vi "Configure Channel.vi"(0 "KS EDU-X 1002G in":refnum<class "KS EDU-X 1002G.lvclass">, 1 "Vertical Scale (5.0 V)":dbl=5.0, 2 "Enable Channel (True)":bool=TRUE, 3 "Impedance (0: 1 MOhm)":i32(ring) items=["1 MOhm", "50 Ohm"], 5 "Cluster":T1={"Channel (0: Channel 1)"=0, "Vertical Coupling (1: DC)"=1, "Probe Attenuation (10: 10X)"=10, "Vertical Range (10.0 V/div)"=10.0, "Vertical Offset (0.0 divs)"=0.0, "Bandwidth (0: MAX Bandwidth)"=0} {"Bandwidth (0: MAX Bandwidth)" items=["MAX Bandwidth", "Unlimited"]; "Probe Attenuation (10: 10X)" items=["1"=1, "10"=10, "20"=20, "50"=50, "100"=100, "500"=500, "1000"=1000]; "Vertical Coupling (1: DC)" items=["AC", "DC", "Ground"]; "Channel (0: Channel 1)" items=["Channel 1", "Channel 2", "Channel 3", "Channel 4", "Math", "Reference A", "Reference B", "Reference C", "Reference D"]}, 11 "error in (no error)":errorcluster, 14 "Vertical Setting (1: Vertical Range)":i32(ring)=1 items=["Vertical Scale", "Vertical Range"]) -> (4 "KS EDU-X 1002G out":refnum<class "KS EDU-X 1002G.lvclass">, 15 "error out":errorcluster)   [LabVIEW 2020, in "Oscilloscope.lvlib" / "KS EDU-X 1002G.lvclass"]
uses:
  KS EDU-X 1002G.lvclass
  C:/Users/ronad/Osciloscopio/Osciloscopio DQMH/Libraries/Oscilloscope/Clases/Osciloscopio/Osciloscopio.lvclass
  Clases/Osciloscopio/Osciloscopio.lvclass/Osciloscopio.ctl
  Clases/Osciloscopio/Read COM.vi
  Clases/Osciloscopio/Write COM.vi
  <instrlib>/Agilent 2000 3000 X-Series/Agilent 2000 3000 X-Series.lvlib
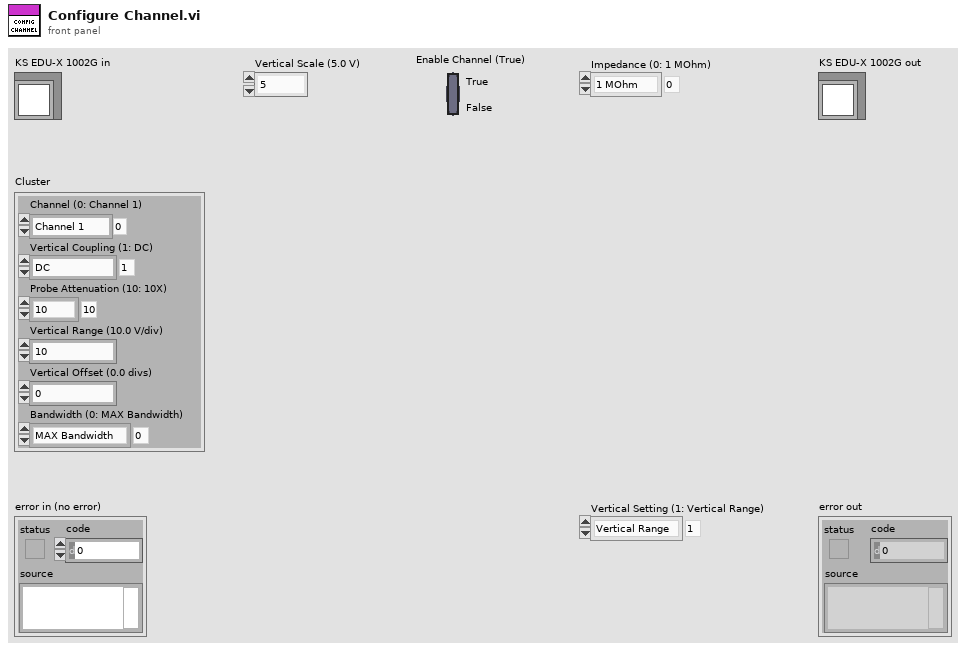
[diagram p1: front panel]
types:
  T1 = cluster{"Channel (0: Channel 1)":i32, "Vertical Coupling (1: DC)":i32, "Probe Attenuation (10: 10X)":i32, "Vertical Range (10.0 V/div)":dbl, "Vertical Offset (0.0 divs)":dbl, "Bandwidth (0: MAX Bandwidth)":i32}
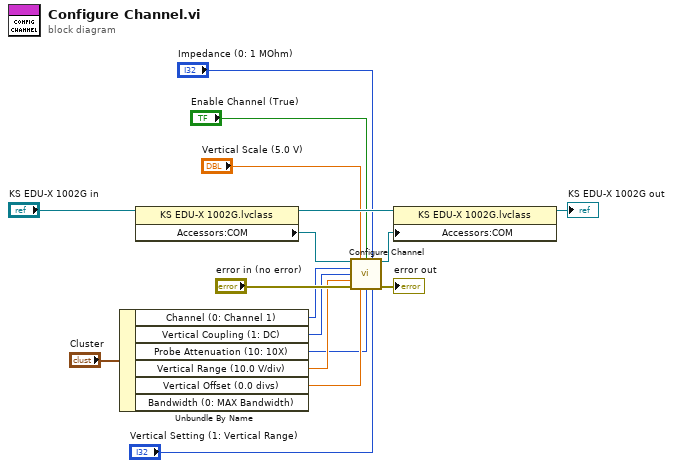
[diagram p0: block diagram]
diagram:
  n1 = Unbundle By Name("Cluster") -> ("Channel (0: Channel 1)"=w8:i32, "Vertical Coupling (1: DC)"=w7:i32, "Probe Attenuation (10: 10X)"=w4:i32, "Vertical Range (10.0 V/div)"=w6:dbl, "Vertical Offset (0.0 divs)"=w5:dbl)  [unwired: 1 out]
  n2 = property class="KS EDU-X 1002G.lvclass"(reference="KS EDU-X 1002G in") -> (reference out=w14:refnum<class "KS EDU-X 1002G.lvclass">, "Accessors:COM"=w16:refnum<visa-resource-name>)  [unwired: 1 in, 1 out]
  n3 = call <instrlib>:"Configure Channel.vi"("VISA resource name"=w16, "Vertical Scale (5.0 V)"="Vertical Scale (5.0 V)", "Enable Channel (T: Enable)"="Enable Channel (True)", "Impedance (0: 1 MOhm)"="Impedance (0: 1 MOhm)", "Channel Name (0: Channel 1)"=w8, "Coupling (1: DC)"=w7, "Vertical Range (40.0 V)"=w6, "error in (no error)"="error in (no error)", "Vertical Offset (0.0)"=w5, "Probe Attenuation (1.0)"=w4, "Vertical Setting (1: Vertical Range)"="Vertical Setting (1: Vertical Range)") -> ("VISA resource name out"=w15:refnum<visa-resource-name>, "error out"=→"error out":errorcluster)  [unwired: 3 in]
  n4 = property class="KS EDU-X 1002G.lvclass"(reference=w14, "Accessors:COM"=w15) -> (reference out=→"KS EDU-X 1002G out":refnum<class "KS EDU-X 1002G.lvclass">)  [unwired: 1 in, 1 out]
